vi "Python_Path_tutorial_3.vi"() -> (3 "appended path":path)   [LabVIEW 2022 SP3]
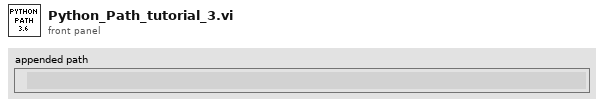
[diagram p1: front panel]
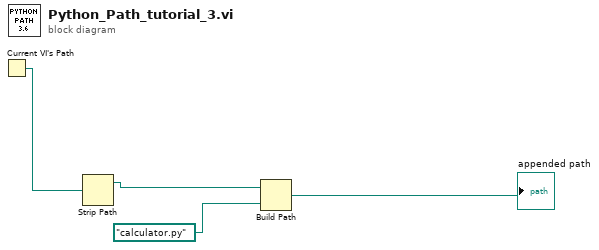
[diagram p0: block diagram]
diagram:
  n1 = Current VI's Path() -> (path=w4:path)
  n2 = Strip Path(path=w4) -> (stripped path=w3:path)  [unwired: 1 out]
  n3 = Build Path(base path=w3, name or relative path=path "calculator.py" ("appended path")) -> (appended path=→"appended path":path)
